vi "Averaging 2.0.vi"(0 "Shorter Name":string, 1 "Timepoints":dbl[](array[numeric]), 2 "Folder to Save":path, 3 "Vy array":dbl[](array[numeric]), 4 "Vx array":dbl[](array[numeric]), 5 "Name of File":string, 6 "Folder Name":string) -> ()   [LabVIEW 2014]
uses:
  <vilib>/Utility/file.llb/Write Delimited Spreadsheet (DBL).vi
  <vilib>/Utility/file.llb/Read Delimited Spreadsheet (DBL).vi
panel:
  out "Diagnostic indicator":dbl
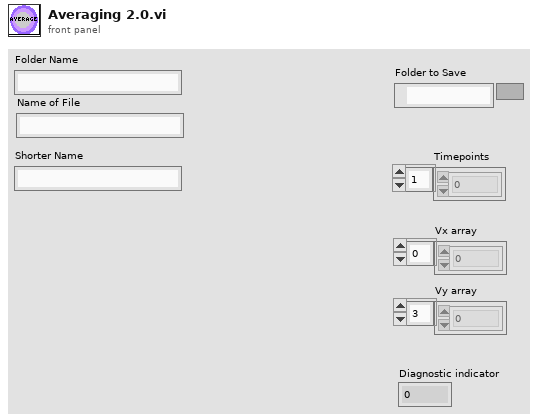
[diagram p1: front panel]
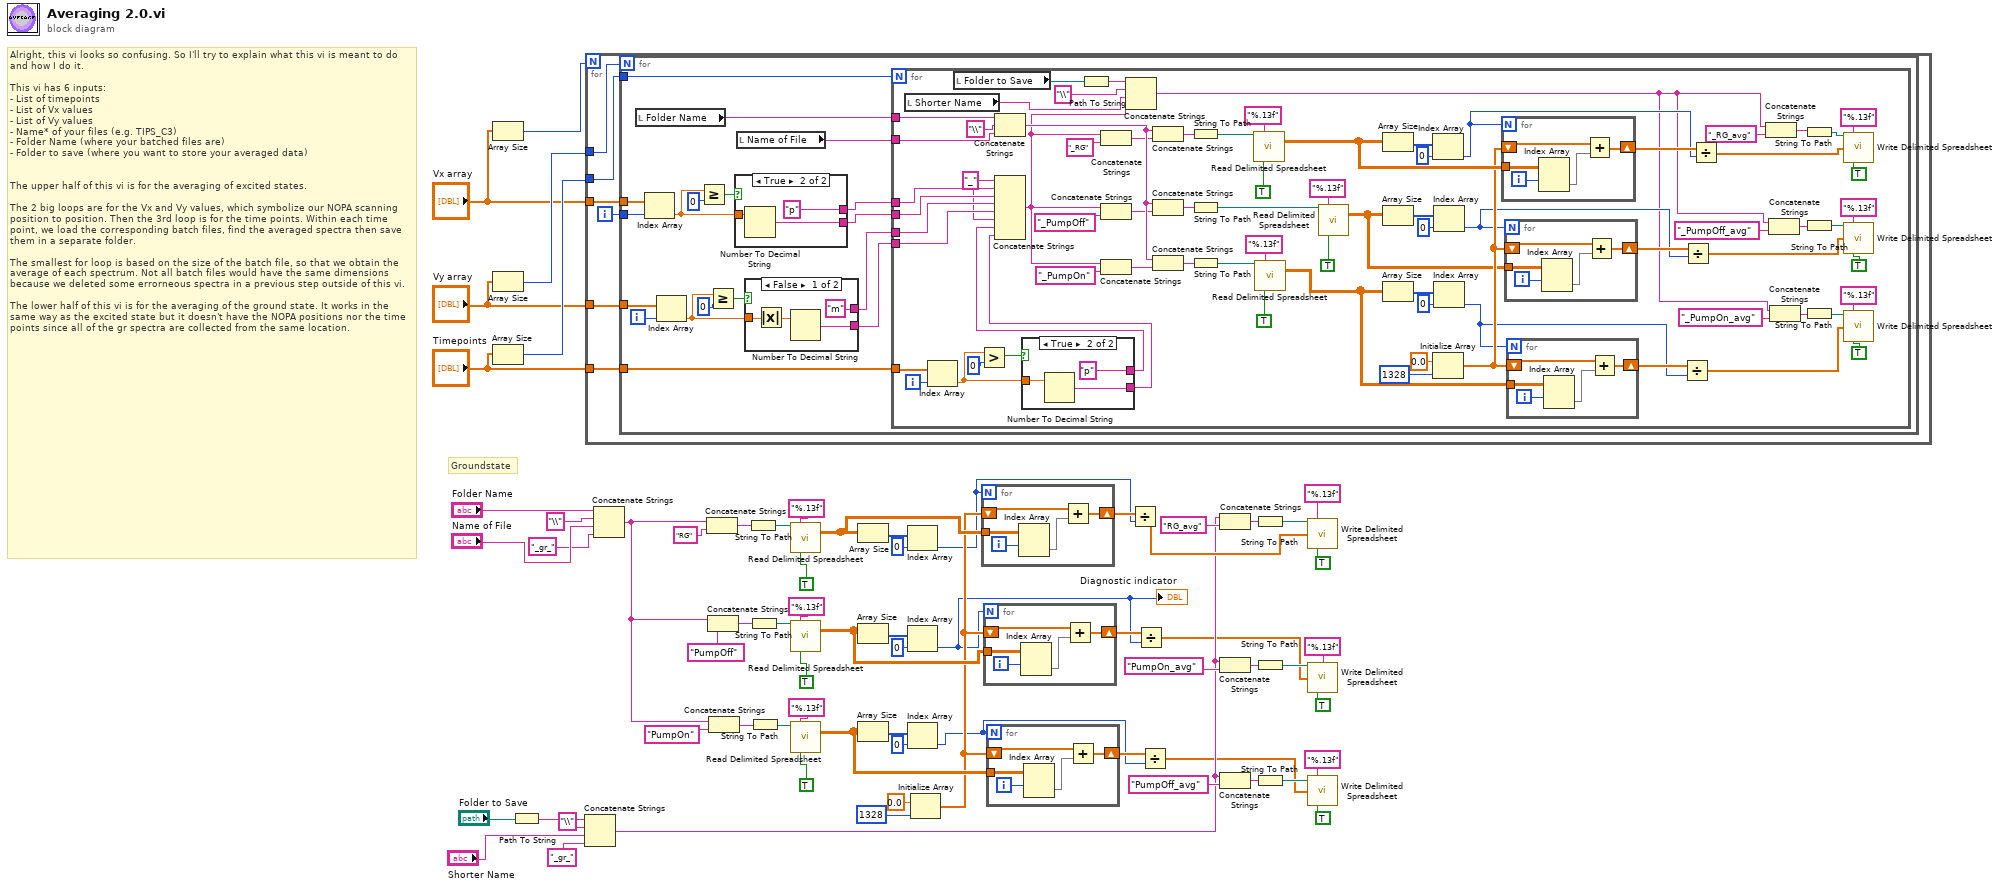
[diagram p0: block diagram]
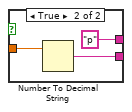
[diagram p2: hidden frame]
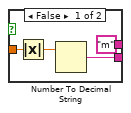
[diagram p3: hidden frame]
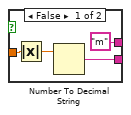
[diagram p4: hidden frame]
diagram:
  # "Groundstate"
  # "Alright, this vi looks so confusing. So I'll try to explain what this vi is meant to do and how I do it.\n\nThis vi has 6 inputs:\n- List of timepoints \n- List of Vx values \n- List of Vy values\n- Name* of your files (e.g. TIPS_C3)\n- Folder Name (where your batched files are)\n- Folder to save (where you want to store your averaged data)\n\n\nThe upper half of this vi is for the averaging of excited states.\n\nThe 2 big loops are for the Vx and Vy values, which symbolize our NOPA scanning position to position. Then the 3rd loop is for the time points. Within each time point, we load the corresponding batch files, find the averaged spectra then save them in a separate folder. \n\nThe smallest for loop is based on the size of the batch file, so that we obtain the average of each spectrum. Not all batch files would have the same dimensions because we deleted some errorneous spectra in a previous step outside of this vi.\n\nThe lower half of this vi is for the averaging of the ground state. It works in the same way as the excited state but it doesn't have the NOPA positions nor the time points since all of the gr spectra are collected from the same location."
  n1 = Array Size(array="Vx array") -> (size(s)=w62:i32)
  n2 = Array Size(array="Vy array") -> (size(s)=w68:i32)
  n3 = Array Size(array="Timepoints") -> (size(s)=w67:i32)
  n4 = Path To String(path="Folder to Save") -> (string=w42:string)
  n5 = Concatenate Strings(w42, "\\" ("string"), "Shorter Name", "_gr_" ("string")) -> (w5:string)
  n6 = for {
    N: w62 -> [_]
    tunnel: w68 -> [w69]
    tunnel: w67 -> [w74]
    tunnel: "Vx array" -> [w73]
    tunnel: "Vy array" -> [w71]
    tunnel: "Timepoints" -> [w70]
    i -> [w72]
    n7 = for {
      N: w69 -> [_]
      tunnel: w74 -> [w92]
      tunnel: w73 -> [w88]
      tunnel: w72 -> [w89]
      tunnel: w71 -> [w84]
      tunnel: w70 -> [w78]
      i -> [w83]
      n8 = local read "Folder Name"() -> (w76:string)
      n9 = Index Array(array=w88, index=w89) -> (element=w77:dbl)
      n10 = Index Array(array=w84, index=w83) -> (element=w85:dbl)
      n11 = Greater Or Equal?(x=w77, y=0) -> (x >= y?=w90:bool)
      n12 = Greater Or Equal?(x=w85, y=0) -> (x >= y?=w87:bool)
      n13 = case shown="True" w90 {
        tunnel: ["m" "p"] -> w82
        tunnel: w77 -> [w103 w104]
        tunnel: [w101 w105] -> w81
        frame False {
          n14 = Absolute Value(x=w103) -> (abs(x)=w102:dbl)
          n15 = Number To Decimal String(number=w102) -> (decimal integer string=w101:string)  [unwired: 1 in]
        }
        frame True {
          n16 = Number To Decimal String(number=w104) -> (decimal integer string=w105:string)  [unwired: 1 in]
        }
      }
      n17 = local read "Name of File"() -> (w75:string)
      n18 = case shown="False" w87 {
        tunnel: ["m" "p"] -> w80
        tunnel: w85 -> [w95 w97]
        tunnel: [w93 w98] -> w79
        frame False {
          n19 = Absolute Value(x=w95) -> (abs(x)=w94:dbl)
          n20 = Number To Decimal String(number=w94) -> (decimal integer string=w93:string)  [unwired: 1 in]
        }
        frame True {
          n21 = Number To Decimal String(number=w97) -> (decimal integer string=w98:string)  [unwired: 1 in]
        }
      }
      n22 = for {
        N: w92 -> [_]
        tunnel: w75 -> [w108]
        tunnel: w76 -> [w182]
        tunnel: w82 -> [w181]
        tunnel: w81 -> [w165]
        tunnel: w80 -> [w180]
        tunnel: w79 -> [w179]
        tunnel: w78 -> [w175]
        i -> [w174]
        w161 = "_"
        n23 = local read "Shorter Name"() -> (w107:string)
        n24 = Index Array(array=w175, index=w174) -> (element=w177:dbl)
        n25 = local read "Folder to Save"() -> (w117:path)
        n26 = Greater?(x=w177, y=0) -> (0:w176:bool)
        n27 = Concatenate Strings(w182, "\\" ("string"), w108) -> (w157:string)
        n28 = case shown="True" w176 {
          tunnel: ["m" "p"] -> w172
          tunnel: w177 -> [w200 w202]
          tunnel: [w198 w203] -> w173
          frame False {
            n29 = Absolute Value(x=w200) -> (abs(x)=w199:dbl)
            n30 = Number To Decimal String(number=w199) -> (decimal integer string=w198:string)  [unwired: 1 in]
          }
          frame True {
            n31 = Number To Decimal String(number=w202) -> (decimal integer string=w203:string)  [unwired: 1 in]
          }
        }
        n32 = Concatenate Strings(w161, w181, w165, w180, w179, w161, w172, w173) -> (w109:string)
        n33 = Path To String(path=w117) -> (string=w116:string)
        n34 = Concatenate Strings(w109, "_RG" ("string")) -> (w155:string)
        n35 = Concatenate Strings(w109, "_PumpOff" ("string")) -> (w151:string)
        n36 = Concatenate Strings(w109, "_PumpOn" ("string")) -> (w152:string)
        n37 = Concatenate Strings(w116, "\\" ("string"), w107, w109) -> (w113:string)
        n38 = Concatenate Strings(w157, w155) -> (w162:string)
        n39 = Concatenate Strings(w157, w151) -> (w159:string)
        n40 = Concatenate Strings(w157, w152) -> (w158:string)
        n41 = String To Path(string=w162) -> (path=w163:path)
        n42 = String To Path(string=w159) -> (path=w146:path)
        n43 = String To Path(string=w158) -> (path=w145:path)
        n44 = call-poly <vilib>:"Read Delimited Spreadsheet.vi"("file path (dialog if empty)"=w163, "format (%.3f)"="%.13f", "transpose? (F)"=TRUE) -> ("all rows"=w133:dbl[][])  [unwired: 7 in, 5 out]
        n45 = call-poly <vilib>:"Read Delimited Spreadsheet.vi"("file path (dialog if empty)"=w145, "format (%.3f)"="%.13f", "transpose? (F)"=TRUE) -> ("all rows"=w128:dbl[][])  [unwired: 7 in, 5 out]
        n46 = call-poly <vilib>:"Read Delimited Spreadsheet.vi"("file path (dialog if empty)"=w146, "format (%.3f)"="%.13f", "transpose? (F)"=TRUE) -> ("all rows"=w127:dbl[][])  [unwired: 7 in, 5 out]
        n47 = Array Size(array=w133) -> (size(s)=w141:i32[])
        n48 = Array Size(array=w127) -> (size(s)=w137:i32[])
        n49 = Array Size(array=w128) -> (size(s)=w136:i32[])
        n50 = Index Array(array=w141, index=0) -> (element=w131:i32)
        n51 = Initialize Array(0.0 ("element"), 1328 ("dimension size")) -> (w129:dbl[])
        n52 = Index Array(array=w137, index=0) -> (element=w124:i32)
        n53 = Index Array(array=w136, index=0) -> (element=w123:i32)
        n54 = for {
          N: w131 -> [_]
          tunnel: w133 -> [w196]
          shift-right: [w193] -> w132
          shift-left: w129 -> [w194]
          i -> [w197]
          n55 = Index Array(array=w196, index (row)=w197) -> (element=w195:dbl[])  [unwired: 1 in]
          n56 = Add(x=w194, y=w195) -> (x+y=w193:dbl[])
        }
        n57 = for {
          N: w124 -> [_]
          tunnel: w127 -> [w191]
          shift-right: [w188] -> w125
          shift-left: w129 -> [w189]
          i -> [w192]
          n58 = Index Array(array=w191, index (row)=w192) -> (element=w190:dbl[])  [unwired: 1 in]
          n59 = Add(x=w189, y=w190) -> (x+y=w188:dbl[])
        }
        n60 = for {
          N: w123 -> [_]
          tunnel: w128 -> [w186]
          shift-right: [w183] -> w126
          shift-left: w129 -> [w184]
          i -> [w187]
          n61 = Index Array(array=w186, index (row)=w187) -> (element=w185:dbl[])  [unwired: 1 in]
          n62 = Add(x=w184, y=w185) -> (x+y=w183:dbl[])
        }
        n63 = Divide(x=w126, y=w123) -> (x/y=w121:dbl[])
        n64 = Divide(x=w125, y=w124) -> (x/y=w122:dbl[])
        n65 = Divide(x=w132, y=w131) -> (x/y=w130:dbl[])
        n66 = Concatenate Strings(w113, "_RG_avg" ("string")) -> (w120:string)
        n67 = Concatenate Strings(w113, "_PumpOff_avg" ("string")) -> (w115:string)
        n68 = Concatenate Strings(w113, "_PumpOn_avg" ("string")) -> (w114:string)
        n69 = String To Path(string=w120) -> (path=w168:path)
        n70 = String To Path(string=w115) -> (path=w167:path)
        n71 = String To Path(string=w114) -> (path=w166:path)
        n72 = call-poly <vilib>:"Write Delimited Spreadsheet.vi"("file path (dialog if empty)"=w168, "format (%.3f)"="%.13f", "1D data"=w130, "transpose? (F)"=TRUE) -> ()  [unwired: 10 in, 2 out]
        n73 = call-poly <vilib>:"Write Delimited Spreadsheet.vi"("file path (dialog if empty)"=w167, "format (%.3f)"="%.13f", "1D data"=w122, "transpose? (F)"=TRUE) -> ()  [unwired: 10 in, 2 out]
        n74 = call-poly <vilib>:"Write Delimited Spreadsheet.vi"("file path (dialog if empty)"=w166, "format (%.3f)"="%.13f", "1D data"=w121, "transpose? (F)"=TRUE) -> ()  [unwired: 10 in, 2 out]
      }
    }
  }
  n75 = Concatenate Strings("Folder Name", "\\" ("string"), "Name of File", "_gr_") -> (w25:string)
  n76 = Concatenate Strings(w25, "RG" ("string")) -> (w33:string)
  n77 = Concatenate Strings(w25, "PumpOff" ("string")) -> (w39:string)
  n78 = Concatenate Strings(w25, "PumpOn" ("string")) -> (w29:string)
  n79 = String To Path(string=w33) -> (path=w31:path)
  n80 = String To Path(string=w39) -> (path=w37:path)
  n81 = String To Path(string=w29) -> (path=w27:path)
  n82 = call-poly <vilib>:"Read Delimited Spreadsheet.vi"("file path (dialog if empty)"=w31, "format (%.3f)"="%.13f", "transpose? (F)"=TRUE) -> ("all rows"=w15:dbl[][])  [unwired: 7 in, 5 out]
  n83 = call-poly <vilib>:"Read Delimited Spreadsheet.vi"("file path (dialog if empty)"=w37, "format (%.3f)"="%.13f", "transpose? (F)"=TRUE) -> ("all rows"=w14:dbl[][])  [unwired: 7 in, 5 out]
  n84 = call-poly <vilib>:"Read Delimited Spreadsheet.vi"("file path (dialog if empty)"=w27, "format (%.3f)"="%.13f", "transpose? (F)"=TRUE) -> ("all rows"=w13:dbl[][])  [unwired: 7 in, 5 out]
  n85 = Array Size(array=w15) -> (size(s)=w19:i32[])
  n86 = Array Size(array=w14) -> (size(s)=w21:i32[])
  n87 = Array Size(array=w13) -> (size(s)=w17:i32[])
  n88 = Index Array(array=w19, index=0) -> (element=w10:i32)
  n89 = Index Array(array=w21, index=0) -> (element=w2:i32)
  "Diagnostic indicator" <- w2
  n90 = Index Array(array=w17, index=0) -> (element=w7:i32)
  n91 = Initialize Array(0.0 ("element"), 1328 ("dimension size")) -> (w12:dbl[])
  n92 = for {
    N: w10 -> [_]
    tunnel: w15 -> [w208]
    shift-right: [w205] -> w11
    shift-left: w12 -> [w206]
    i -> [w209]
    n93 = Index Array(array=w208, index (row)=w209) -> (element=w207:dbl[])  [unwired: 1 in]
    n94 = Add(x=w206, y=w207) -> (x+y=w205:dbl[])
  }
  n95 = for {
    N: w2 -> [_]
    tunnel: w14 -> [w213]
    shift-right: [w210] -> w9
    shift-left: w12 -> [w211]
    i -> [w214]
    n96 = Index Array(array=w213, index (row)=w214) -> (element=w212:dbl[])  [unwired: 1 in]
    n97 = Add(x=w211, y=w212) -> (x+y=w210:dbl[])
  }
  n98 = for {
    N: w7 -> [_]
    tunnel: w13 -> [w218]
    shift-right: [w215] -> w8
    shift-left: w12 -> [w216]
    i -> [w219]
    n99 = Index Array(array=w218, index (row)=w219) -> (element=w217:dbl[])  [unwired: 1 in]
    n100 = Add(x=w216, y=w217) -> (x+y=w215:dbl[])
  }
  n101 = Divide(x=w11, y=w10) -> (x/y=w6:dbl[])
  n102 = Divide(x=w9, y=w2) -> (x/y=w4:dbl[])
  n103 = Divide(x=w8, y=w7) -> (x/y=w3:dbl[])
  n104 = Concatenate Strings(w5, "RG_avg") -> (w48:string)
  n105 = Concatenate Strings(w5, "PumpOn_avg") -> (w49:string)
  n106 = Concatenate Strings(w5, "PumpOff_avg") -> (w50:string)
  n107 = String To Path(string=w48) -> (path=w52:path)
  n108 = String To Path(string=w49) -> (path=w54:path)
  n109 = String To Path(string=w50) -> (path=w56:path)
  n110 = call-poly <vilib>:"Write Delimited Spreadsheet.vi"("file path (dialog if empty)"=w52, "format (%.3f)"="%.13f", "1D data"=w6, "transpose? (F)"=TRUE) -> ()  [unwired: 10 in, 2 out]
  n111 = call-poly <vilib>:"Write Delimited Spreadsheet.vi"("file path (dialog if empty)"=w54, "format (%.3f)"="%.13f", "1D data"=w4, "transpose? (F)"=TRUE) -> ()  [unwired: 10 in, 2 out]
  n112 = call-poly <vilib>:"Write Delimited Spreadsheet.vi"("file path (dialog if empty)"=w56, "format (%.3f)"="%.13f", "1D data"=w3, "transpose? (F)"=TRUE) -> ()  [unwired: 10 in, 2 out]
